vi "VCS Get Master Encoder Parameter.vi"(3 "error in (no error)":errorcluster, 5 "axis in":cluster{"keyHandle":u32, "nodeId":u16}={"keyHandle"=0, "nodeId"=1}) -> (0 "error out":errorcluster, 1 "master encoder parameter":T1, 2 "axis out":cluster{"keyHandle":u32, "nodeId":u16}={"keyHandle"=0, "nodeId"=1})   [LabVIEW 2017, in "maxonEPOS.lvlib"]
doc: "With function „VCS_GetMasterEncoderParameter” it is possible to read all parameters for master encoder mode."
uses:
  Examples/maxonEPOS.lvlib
  SSI_Tool/InstrumentsInterfaces/Motordriver/maxon EPOS/Resources/EposCmd.dll
  SSI_Tool/InstrumentsInterfaces/Motordriver/maxon EPOS/Resources/EposCmd64.dll
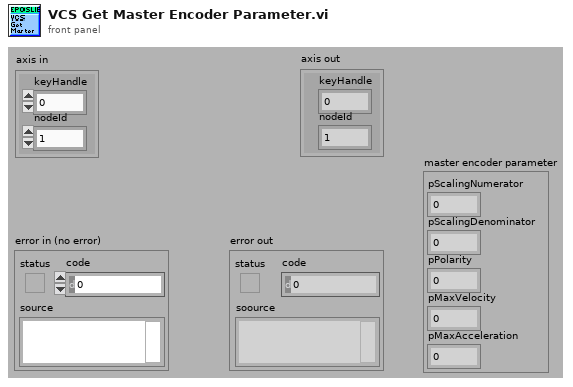
[diagram p1: front panel]
types:
  T1 = cluster{"pScalingNumerator":u16, "pScalingDenominator":u16, "pPolarity":u8, "pMaxVelocity":u32, "pMaxAcceleration":u32}
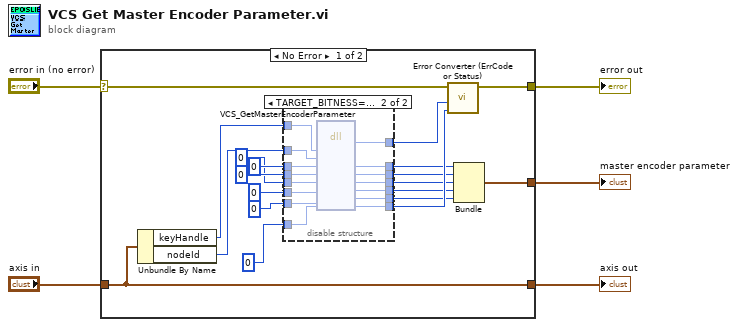
[diagram p0: block diagram]
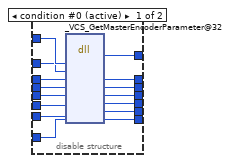
[diagram p2: hidden frame]
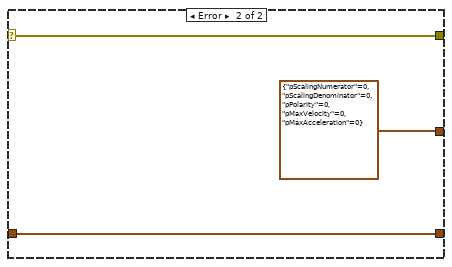
[diagram p3: hidden frame]
diagram:
  n1 = case shown="No Error" "error in (no error)" {
    selector: "error in (no error)" -> [w22 w56]
    tunnel: "axis in" -> [w24 w57]
    tunnel: [w24 w57] -> w4
    tunnel: [w23 w56] -> w3
    tunnel: [w11 T1 {"pScalingNumerator"=0, "pScalingDenominator"=0, "pPolarity"=0, "pMaxVelocity"=0, "pMaxAcceleration"=0}] -> w1
    frame No Error {
      n2 = Unbundle By Name(w24) -> ("keyHandle"=w20:u32, "nodeId"=w19:u16)
      n3 = disable-structure shown="TARGET_BITNESS==64" {
        disable-tunnel: u32 0 ("pErrorCode") -> [w39 w54]
        disable-tunnel: w20 -> [w38 w53]
        disable-tunnel: w19 -> [w37 w52]
        disable-tunnel: [w36 w51] -> w18
        disable-tunnel: [w35 w50] -> w17
        disable-tunnel: [w34 w49] -> w16
        disable-tunnel: [w33 w48] -> w15
        disable-tunnel: [w32 w47] -> w14
        disable-tunnel: [w31 w46] -> w13
        disable-tunnel: [w30 w45] -> w12
        disable-tunnel: u16 0 ("pScalingNumerator") -> [w29 w44]
        disable-tunnel: u16 0 ("pScalingDenominator") -> [w28 w43]
        disable-tunnel: u8 0 ("pPolarity") -> [w27 w42]
        disable-tunnel: u32 0 ("pMaxVelocity") -> [w26 w41]
        disable-tunnel: u32 0 ("pMaxAcceleration") -> [w25 w40]
        frame condition #0 (active) {
          n4 = dll-call lib="C:/workspace/project/scancon/sw/SSI_Tool/InstrumentsInterfaces/Motordriver/maxon EPOS/Resources/EposCmd.*" fn="_VCS_GetMasterEncoderParameter@32"("KeyHandle"=w38, "NodeId"=w37, "pScalingNumerator"=w29, "pScalingDenominator"=w28, "pPolarity"=w27, "pMaxVelocity"=w26, "pMaxAcceleration"=w25, "pErrorCode"=w39) -> ("Rückgabetyp"=w36:i32, "pScalingNumerator"=w34:u16, "pScalingDenominator"=w33:u16, "pPolarity"=w32:u8, "pMaxVelocity"=w31:u32, "pMaxAcceleration"=w30:u32, "pErrorCode"=w35:u32)  [unwired: 5 in, 2 out]
        }
        frame condition #1 {
          n5 = dll-call lib="C:/Sources/LabVIEW/maxon EPOS/Resources/EposCmd64.*" fn="VCS_GetMasterEncoderParameter" ("EposCmd.dll:_VCS_GetMasterEncoderParameter@32")("KeyHandle"=w53, "NodeId"=w52, "pScalingNumerator"=w44, "pScalingDenominator"=w43, "pPolarity"=w42, "pMaxVelocity"=w41, "pMaxAcceleration"=w40, "pErrorCode"=w54) -> ("Rückgabetyp"=w51:i32, "pScalingNumerator"=w49:u16, "pScalingDenominator"=w48:u16, "pPolarity"=w47:u8, "pMaxVelocity"=w46:u32, "pMaxAcceleration"=w45:u32, "pErrorCode"=w50:u32)  [unwired: 5 in, 2 out]
        }
      }
      n6 = call "Error Converter (ErrCode or Status).vi"("error code"=w17, "return type"=w18, "error in (no error)"=w22) -> ("error out"=w23:errorcluster)  [unwired: 7 in]
      n7 = Bundle("pScalingNumerator"=w16, "pScalingDenominator"=w15, "pPolarity"=w14, "pMaxVelocity"=w13, "pMaxAcceleration"=w12) -> (w11:T1)  [unwired: 1 in]
    }
    frame Error {
    }
  }
  "error out" <- w3
  "axis out" <- w4
  "master encoder parameter" <- w1
